vi "getChannelType.vi"(8 "error in (no error)":errorcluster, 11 "DeviceData in":refnum<class "DeviceData.lvclass">) -> (0 "error out":errorcluster, 2 "type":T1(ring), 3 "DeviceData out":refnum<class "DeviceData.lvclass">)   [LabVIEW 2009, in "DataMappers.lvlib" / "DeviceData.lvclass"]
uses:
  DeviceData.lvclass
  DeviceData.lvclass/DeviceData.ctl
  DatabaseHelpers/Database Objects/device/device.lvclass
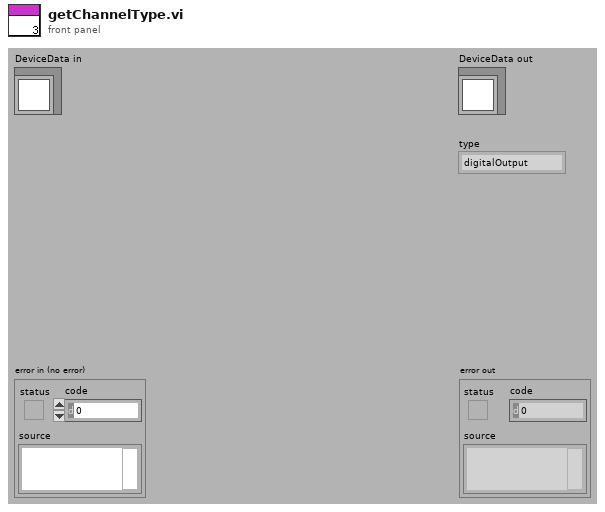
[diagram p1: front panel]
types:
  T1 = enum16{"digitalOutput", "digitalInput", "analogOutput", "analogInput", "rfOutput", "ethernetSupply"}
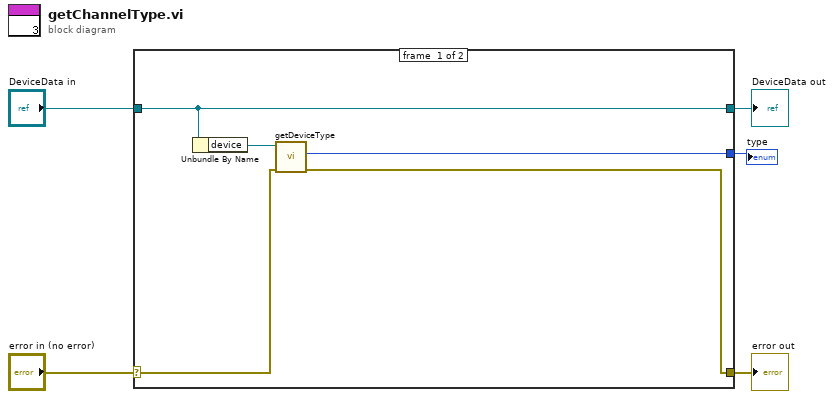
[diagram p0: block diagram]
diagram:
  n1 = case shown="No Error" "error in (no error)" {
    selector: "error in (no error)" -> [w8 w12]
    tunnel: [w7 w12] -> w4
    tunnel: [w10 w11] -> w2
    tunnel: "DeviceData in" -> [w10 w11]
    tunnel: [w6 _] -> w1
    frame #0 {
      n2 = Unbundle By Name(w10) -> ("device"=w9:refnum<class "device.lvclass">)
      n3 = call-dynamic "getDeviceType.vi"("error in (no error)"=w8, "device.lvclass in"=w9) -> ("error out"=w7:errorcluster, "type"=w6:T1)  [unwired: 7 in, 1 out]
    }
    frame #1 {
    }
  }
  "error out" <- w4
  "DeviceData out" <- w2
  "type" <- w1
